vi "Save Moving Image.vi"() -> ()   [LabVIEW 2017]
uses:
  IMAQCV/PIIO/Core/PIIO DIO.ctl
  IMAQCV/GPIO/GPIO Pins.ctl
  <vilib>/Platform/TimedLoop/XDataNode/timing_clust.ctl
  <vilib>/Platform/TimedLoop/XDataNode/nitl_modes.ctl
  <vilib>/Platform/TimedLoop/XDataNode/wakeup.ctl
  <vilib>/platform/TimedLoop/XDataNode/XDataNode.xnode
  IMAQCV/PIIO.lvlib
  IMAQCV/IMAQCV.lvlib
  IMAQCV/LVOpenCV.lvlib
  <vilib>/Platform/TimedLoop/XDataNode/XDNodeRunTimeDep.lvlib
panel:
  in  "PIN":T1 items=["L1", "L2"]
  in  "delay (ms)":u32=150
  out "moving time (ms)":u32
  in  "LED Flash":bool
  in  "LED":bool
  in  "Gain (0=auto)":i32(slide) scale=0.0..100.0
  in  "Brightness":i32(slide)=50 scale=0.0..100.0
  in  "Contrast":i32(slide)=50 scale=0.0..100.0
  in  "Saturation":i32(slide)=50 scale=0.0..100.0
  in  "Sharpness":i32(slide)=50 scale=0.0..100.0
  in  "Rotation":i32(ring) items=["0", "90", "180", "270"]
  in  "Flip Horizontal":bool
  in  "Flip Vertical":bool
  in  "AWB":T2(ring)
  in  "Meter":enum16{"AVERAGE", "SPOT", "BACKLIT", "MATRIX"}(ring)
  in  "Effect":T3(ring)
  in  "Shutter (us, 0=auto)":i32
  out "output per minute":u32
  in  "File Format":string="camera-%03d.jpg"
  in  "Enable Save Files":bool
  in  "Image Index":u32
  in  "Image File Path":path=path "c:/project-01/camera-000.jpg"
  in  "FPS":i32=30
  in  "RGB LED 8x8":u32[][](array[colorbox])=[[0, 0, 16777215, 16777215, 16777215, 16777215, 16777215, 16777215], [0, 16777215, 16777215, 16777215, 16777215, 16777215, 16777215, 16777215], [16777215, 16777215, 16777215, 16777215, 16777215, 16777215, 16777215, 16777215], [16777215, 16777215, 0, 0, 0, 0, 0, 0], [16777215, 16777215, 0, 0, 0, 0, 0, 0], [16777215, 16777215, 0, 0, 0, 0, 0, 0], [16777215, 16777215, 0, 0, 0, 0, 0, 0], [0, 16777215, 16777215, 16777215, 16777215, 0, 0, 0]]
  in  "Image Size":T4(ring)=enum."640 (H)   x  480 (V) "
  out "picture":picture
  out "image processing time (ms)":u32
  out "DI-CH4":bool
  out "DI-CH2":bool
  out "DI-CH3":bool
  out "DI-CH1":bool
  in  "stop":bool
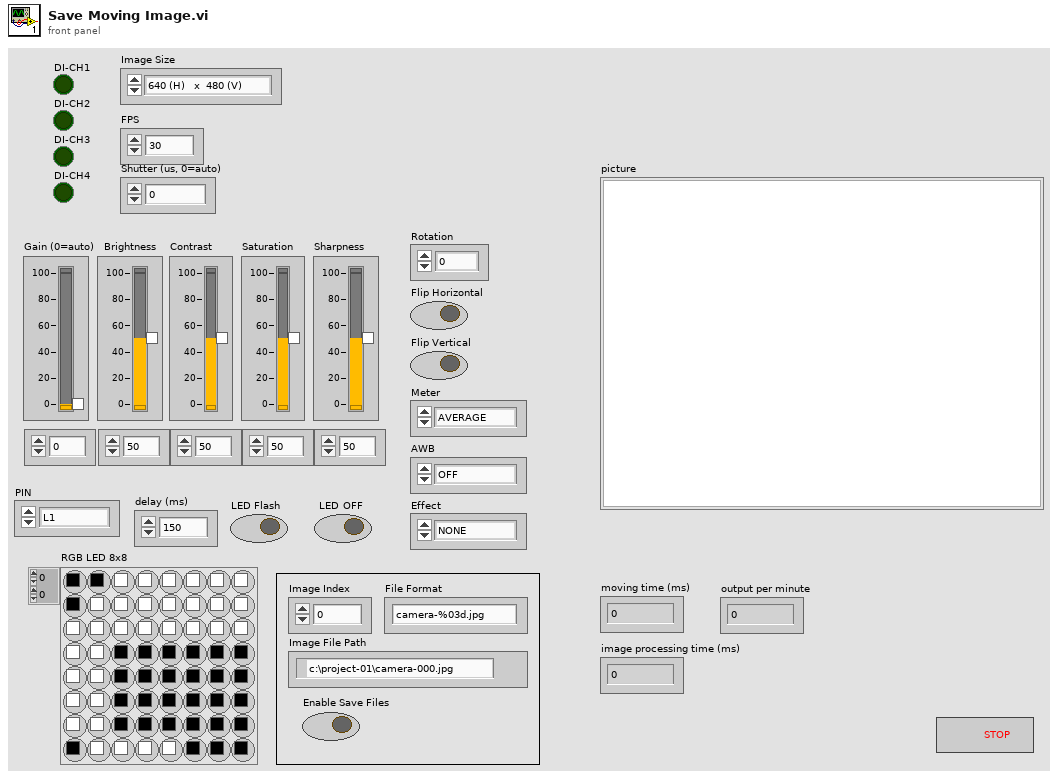
[diagram p1: front panel]
types:
  T1 = typedef "PIIO.lvlib/PIIO DIO.ctl" = u8
  T2 = enum16{"OFF", "AUTO", "SUNLIGHT", "CLOUDY", "SHADE", "TUNGSTEN", "FLUORESCENT", "INCANDESCENT", "FLASH"}
  T3 = enum16{"NONE", "NEGATIVE", "SOLARIZE", "SKETCH", "DENOISE", "EMBOSS", "OILPAINT", "HATCH", "GPEN", "PASTEL", "WATERCOLOR", "FILM", "BLUR", "SATURATION", "COLORSWAP", "WASHEDOUT", "POSTERISE", "COLORPOINT", "COLORBALANCE", "CARTOON"}
  T4 = enum16{"320 (H)   x  240 (V)", "352(H)    x  288 (V)", "640 (H)   x  480 (V) ", "800 (H)   x  600 (V)", "1024 (H) x  768 (V)", "1280 (H) x  720 (V)", "1280 (H) x  960 (V)", "1280 (H) x 1024 (V)", "1920 (H) x 1080 (V)"}
  T5 = typedef "PIIO.lvlib/GPIO Pins.ctl" = u8
  T6 = cluster{"GPIO":T5[], "MODE":enum8{"INPUT", "OUTPUT", "PWM_OUTPUT", "GPIO_CLOCK", "SOFT_PWM_OUTPUT", "SOFT_TONE_OUTPUT", "PWM_TONE_OUTPUT"}[]}
  T7 = typedef "Image Type" = u32
  T8 = typedef "IMAQCV.lvlib/IMAQCV Image.ctl" = refnum<vi>
  T9 = typedef "XDNodeRunTimeDep.lvlib/timing_clust.ctl" = cluster{"Expected End [f-1]":u64, "Actual End [f-1]":u64, "Finished Late? [f-1]":bool, "Expected End [i-1]":u64, "Actual End [i-1]":u64, "Finished Late? [i-1]":bool, "Expected Start [i]":u64, "Actual Start [i]":u64, "Expected Start [f]":u64, "Actual Start [f]":u64, "Source Name":string, "Structure Name":string, "Period":i64, "Deadline":i64, "Offset":i64, "Start":i64, "Priority":i32, "Timeout":i32, "Mode":T10, "Wakeup Reason":T11, "Error":errorcluster, "Source Type":string, "Secondary Source Type":string, "Global End Time":u64, "Global Start Time":u64, "Frame Duration":u64, "Iteration Duration":u64, "Assigned CPU":i32, "I/O Scan Engine Mode":u32}
  T10 = typedef "XDNodeRunTimeDep.lvlib/nitl_modes.ctl" = enum32{"No Change", "Process missed periods, maintain original phase", "Discard missed periods, maintain original phase", "Process missed periods, ignore original phase", "Discard missed periods, ignore original phase"}
  T11 = typedef "XDNodeRunTimeDep.lvlib/wakeup.ctl" = enum32{"Normal", "Aborted", "Asynchronous wakeup", "Timing source error", "Timed loop error", "Timeout"}
  T12 = typedef "IMAQ Image.ctl" = refnum<image>
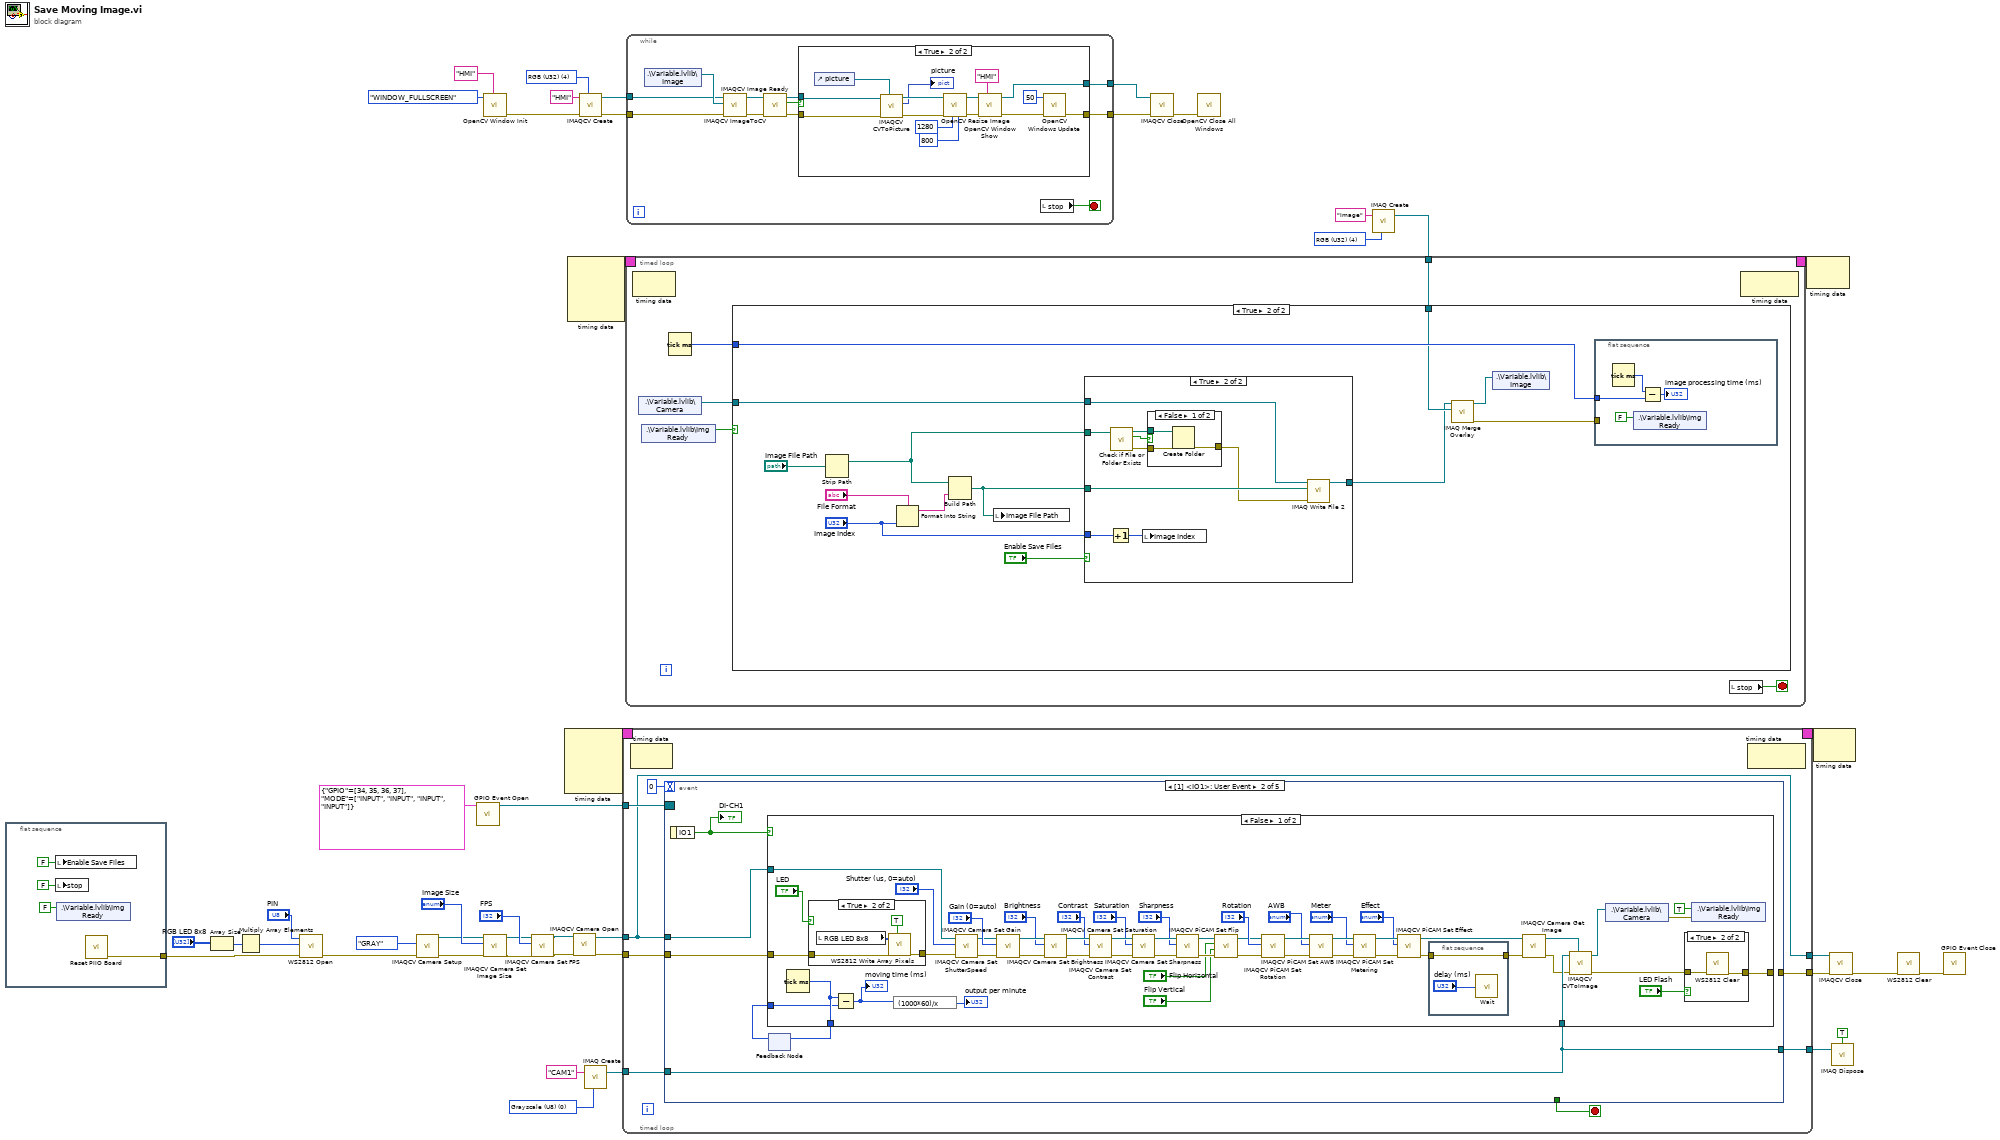
[diagram p0: block diagram]
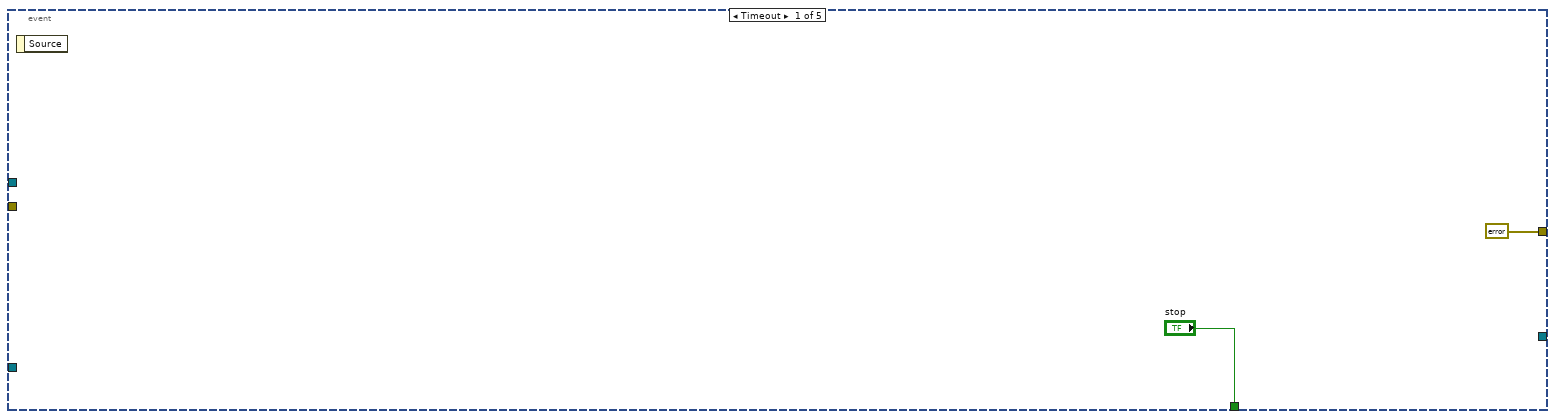
[diagram p6: hidden frame]
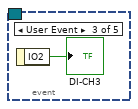
[diagram p10: hidden frame]
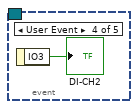
[diagram p11: hidden frame]
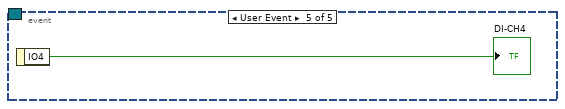
[diagram p12: hidden frame]
diagram:
  w20 = T7 4 items=["Grayscale (U8)", "Grayscale (I16)", "Grayscale (SGL)", "Complex (CSG)", "RGB (U32)", "HSL (U32)", "RGB (U64)", "Grayscale (U16)"] ("Image Type")
  w31 = u32 4 items=["Grayscale (U8)", "Grayscale (I16)", "Grayscale (SGL)", "Complex (CSG)", "RGB (U32)", "HSL (U32)", "RGB (U64)", "Grayscale (U16)"] ("Image Type")
  w36 = T7 0 items=["Grayscale (U8)", "Grayscale (I16)", "Grayscale (SGL)", "Complex (CSG)", "RGB (U32)", "HSL (U32)", "RGB (U64)", "Grayscale (U16)"] ("Image Type")
  n1 = flat-sequence {
    tunnel: [w47] -> w12
    frame #0 {
      n2 = local write "Enable Save Files"(FALSE ("Enable Save Files")) -> ()
      n3 = local write "stop"(FALSE ("stop")) -> ()
      n4 = shared-variable ".\\Variable.lvlib\\Img Ready"(FALSE ("outReady")) -> ()  [unwired: 1 in, 1 out]
      n5 = call "Reset PIIO Board.vi"() -> ("error out"=w47:errorcluster)  [unwired: 11 in]
    }
  }
  n6 = Array Size(array="RGB LED 8x8") -> (size(s)=w11:i32[])
  n7 = Multiply Array Elements(1:w11) -> (0:w9:i32)
  n8 = call "WS2812 Open.vi"("Error In"=w12, "Number of LEDs"=w9, "PIN"="PIN") -> ("Error Out"=w25:errorcluster)  [unwired: 8 in]
  n9 = call "IMAQCV Camera Setup.vi"("error in (no error)"=w25, "type"=enum16{"GRAY", "COLOR"}."GRAY") -> ("error out"=w26:errorcluster, "image out"=w27:T8)  [unwired: 8 in]
  n10 = call "GPIO Event Open.vi"("GPIO"=T6 {"GPIO"=[34, 35, 36, 37], "MODE"=[enum."INPUT", enum."INPUT", enum."INPUT", enum."INPUT"]}) -> ("Event Registration Refnum"=w13:refnum<event-registration>)  [unwired: 9 in, 1 out]
  n11 = call "OpenCV Window Init.vi"("window name"="HMI", "mode"=enum8{"WINDOW_AUTOSIZE", "WINDOW_FULLSCREEN"}."WINDOW_FULLSCREEN") -> ("error out"=w17:errorcluster)  [unwired: 9 in]
  n12 = call "IMAQCV Camera Set Image Size.vi"("error in (no error)"=w26, "Image Size"="Image Size", "image in"=w27) -> ("error out"=w8:errorcluster, "image out"=w7:T8)  [unwired: 7 in]
  n13 = call "IMAQCV Camera Set FPS.vi"("error in (no error)"=w8, "FPS"="FPS", "image in"=w7) -> ("error out"=w6:errorcluster, "image out"=w5:T8)  [unwired: 7 in]
  n14 = node-c288() -> (w45:T9)  [unwired: 4 in]
  n15 = node-c288() -> (w43:T9)  [unwired: 4 in]
  n16 = call "IMAQCV Camera Open.vi"("error in (no error)"=w6, "image in"=w5) -> ("error out"=w16:errorcluster, "image out"=w15:T8)  [unwired: 8 in]
  n17 = call "IMAQCV Create.vi"("Image Type"=w31, "error in (no error)"=w17, "Image Name"="HMI") -> ("error out"=w18:errorcluster, "Image Out"=w19:T8)  [unwired: 7 in]
  n18 = call "IMAQ Create"("Image Name"="CAM1", "Image Type"=w36) -> ("New Image"=w35:T12)  [unwired: 3 in, 1 out]
  n19 = timed-loop {
    tunnel: w13 -> [w55]
    tunnel: [w54] -> w40
    tunnel: w16 -> [w53]
    tunnel: w15 -> [w52]
    tunnel: [w52] -> w38
    tunnel: w35 -> [w51]
    timing: w45 -> [_]
    timing-out: [_] -> w44
    tunnel: [w50] -> w3
    stop <- w57 stop-if-true
    n20 = node-c288() -> ()  [unwired: 1 in, 1 out]
    n21 = event shown="[1] <IO1>: User Event" {
      selector: w55 -> [_ _ _ _ _]
      dyn-events: _ -> [_ _ _ _ _]
      timeout: 0 -> [_ _ _ _ _]
      tunnel: ["stop" _ _ _ _] -> w57
      tunnel: [errorcluster {"status"=FALSE, "code"=0, "source"=""} ("error out") _ _ _ _] -> w54
      tunnel: w52 -> [_ w64 _ _ _]
      tunnel: w53 -> [_ w65 _ _ _]
      tunnel: w51 -> [_ w63 _ _ _]
      tunnel: [_ w63 _ _ _] -> w50
      event Timeout {
        n22 = event-data() -> ()  [unwired: 1 in, 1 out]
      }
      event User Event {
        n23 = event-data() -> ("IO1"=w62:bool)  [unwired: 1 in]
        "DI-CH1" <- w62
        n24 = feedback #1() -> (w67:u32)  [unwired: 1 in]
        n25 = case shown="False" w62 {
          tunnel: w65 -> [w107 w131]
          tunnel: [w118 w131] -> _
          tunnel: w64 -> [w71 _]
          tunnel: w63 -> [w110 _]
          tunnel: w67 -> [w113 w130]
          tunnel: [w114 w130] -> w66
          frame False {
            n26 = Tick Count (ms)() -> (millisecond timer value=w114:u32)
            n27 = case shown="True" "LED" {
              tunnel: w107 -> [w120 w124]
              tunnel: [w120 w121] -> w73
              frame False {
              }
              frame True {
                n28 = local read "RGB LED 8x8"() -> (w122:u32[][])
                n29 = call "WS2812 Write Array Pixels.vi"("Refresh? (True)"=TRUE, "Error In"=w124, "pixmap"=w122) -> ("Error Out"=w121:errorcluster)  [unwired: 8 in]
              }
            }
            n30 = Subtract(x=w114, y=w113) -> (x-y=w69:u32)
            "moving time (ms)" <- w69
            n31 = expression code="(1000*60)/x"(w69) -> (→"output per minute":u32)
            n32 = call "IMAQCV Camera Set ShutterSpeed.vi"("error in (no error)"=w73, "shutter speed (us, 0=auto)"="Shutter (us, 0=auto)", "image in"=w71) -> ("error out"=w76:errorcluster, "image out"=w75:T8)  [unwired: 7 in]
            n33 = call "IMAQCV Camera Set Gain.vi"("error in (no error)"=w76, "gain (0=auto)"="Gain (0=auto)", "image in"=w75) -> ("error out"=w104:errorcluster, "image out"=w105:T8)  [unwired: 7 in]
            n34 = call "IMAQCV Camera Set Brightness.vi"("error in (no error)"=w104, "brightness"="Brightness", "image in"=w105) -> ("error out"=w103:errorcluster, "image out"=w100:T8)  [unwired: 7 in]
            n35 = call "IMAQCV Camera Set Contrast.vi"("error in (no error)"=w103, "contrast"="Contrast", "image in"=w100) -> ("error out"=w102:errorcluster, "image out"=w99:T8)  [unwired: 7 in]
            n36 = call "IMAQCV Camera Set Saturation.vi"("error in (no error)"=w102, "saturation"="Saturation", "image in"=w99) -> ("error out"=w101:errorcluster, "image out"=w98:T8)  [unwired: 7 in]
            n37 = call "IMAQCV Camera Set Sharpness.vi"("error in (no error)"=w101, "sharpness"="Sharpness", "image in"=w98) -> ("error out"=w91:errorcluster, "image out"=w90:T8)  [unwired: 7 in]
            n38 = call "IMAQCV PiCAM Set Flip.vi"("error in (no error)"=w91, "vertical"="Flip Vertical", "horizontal"="Flip Horizontal", "image in"=w90) -> ("error out"=w89:errorcluster, "image out"=w88:T8)  [unwired: 6 in]
            n39 = call "IMAQCV PiCAM Set Rotation.vi"("error in (no error)"=w89, "Rotation"="Rotation", "image in"=w88) -> ("error out"=w85:errorcluster, "image out"=w84:T8)  [unwired: 7 in]
            n40 = call "IMAQCV PiCAM Set AWB.vi"("error in (no error)"=w85, "AWB"="AWB", "image in"=w84) -> ("error out"=w82:errorcluster, "image out"=w80:T8)  [unwired: 7 in]
            n41 = call "IMAQCV PiCAM Set Metering.vi"("error in (no error)"=w82, "mode"="Meter", "image in"=w80) -> ("error out"=w81:errorcluster, "image out"=w79:T8)  [unwired: 7 in]
            n42 = call "IMAQCV PiCAM Set Effect.vi"("error in (no error)"=w81, "effect"="Effect", "image in"=w79) -> ("error out"=w72:errorcluster, "image out"=w70:T8)  [unwired: 7 in]
            n43 = flat-sequence {
              tunnel: [w128] -> w119
              tunnel: w72 -> [w128]
              frame #0 {
                n44 = call "Wait"("Count(mSec)"="delay (ms)") -> ()  [unwired: 1 out]
              }
            }
            n45 = call "IMAQCV Camera Get Image.vi"("error in (no error)"=w119, "image in"=w70) -> ("error out"=w109:errorcluster, "image out"=w108:T8)  [unwired: 8 in]
            n46 = call "IMAQCV CVToImage.vi"("cvimage in"=w108, "error in (no error)"=w109, "Variant In"=w110) -> ("error out"=w115:errorcluster, "Variant Out"=w111:refnum<image>)  [unwired: 7 in]
            n47 = shared-variable ".\\Variable.lvlib\\Camera"(w111) -> (error out=w116:errorcluster)  [unwired: 1 in]
            n48 = case shown="True" "LED Flash" {
              tunnel: [w125 w127] -> w118
              tunnel: w115 -> [w125 w126]
              frame False {
              }
              frame True {
                n49 = call "WS2812 Clear.vi"("Error In"=w126) -> ("Error Out"=w127:errorcluster)  [unwired: 10 in]
              }
            }
            n50 = shared-variable ".\\Variable.lvlib\\Img Ready"(TRUE ("ready"), error in=w116) -> ()  [unwired: 1 out]
          }
          frame True {
          }
        }
        n51 = feedback-in #1(w66) -> ()
      }
      event User Event {
        n52 = event-data() -> ("IO2"=→"DI-CH3":bool)  [unwired: 1 in]
      }
      event User Event {
        n53 = event-data() -> ("IO3"=→"DI-CH2":bool)  [unwired: 1 in]
      }
      event User Event {
        n54 = event-data() -> ("IO4"=→"DI-CH4":bool)  [unwired: 1 in]
      }
    }
    n55 = node-c288() -> ()  [unwired: 1 in, 1 out]
  }
  n56 = while {
    tunnel: [w144] -> w24
    tunnel: [w143] -> w23
    tunnel: w19 -> [w138]
    tunnel: w18 -> [w135]
    stop <- w145 stop-if-true
    n57 = shared-variable ".\\Variable.lvlib\\Image"() -> (w139:refnum<image>)  [unwired: 1 in, 1 out]
    n58 = call "IMAQCV ImageToCV.vi"("error in (no error)"=w135, "Variant In"=w139, "CV in"=w138) -> ("error out"=w136:errorcluster, "CV out"=w137:T8)  [unwired: 7 in]
    n59 = call "IMAQCV Image Ready.vi"("error in (no error)"=w136, "image in"=w137) -> ("error out"=w141:errorcluster, "ready?"=w140:bool, "image out"=w142:T8)  [unwired: 7 in]
    n60 = case shown="True" w140 {
      tunnel: [w146 w159] -> w144
      tunnel: [w147 w158] -> w143
      tunnel: w142 -> [w146 w150]
      tunnel: w141 -> [w147 w151]
      frame False {
      }
      frame True {
        n61 = control-ref of="picture"() -> (w149:refnum<vi>)
        n62 = call "IMAQCV CVToPicture.vi"("picture ref"=w149, "error in (no error)"=w151, "image"=w150) -> ("error out"=w152:errorcluster, "picture"=→"picture":picture, "image out"=w153:T8)  [unwired: 6 in]
        n63 = call "OpenCV Resize Image.vi"("height"=u32 800, "width"=u32 1280, "error in (no error)"=w152, "image in"=w153) -> ("error out"=w154:errorcluster, "image out"=w155:T8)  [unwired: 6 in]
        n64 = call "OpenCV Window Show.vi"("window name"="HMI", "error in (no error)"=w154, "image in"=w155) -> ("error out"=w160:errorcluster, "image out"=w159:T8)  [unwired: 7 in]
        n65 = call "OpenCV Windows Update.vi"("error in (no error)"=w160, "wait ms"=50) -> ("error out"=w158:errorcluster)  [unwired: 8 in, 1 out]
      }
    }
    n66 = local read "stop"() -> (w145:bool)
  }
  n67 = call "IMAQCV Close.vi"("error in (no error)"=w23, "Image"=w24) -> ("error out"=w33:errorcluster)  [unwired: 9 in]
  n68 = call "OpenCV Close All Windows.vi"("error in (no error)"=w33) -> ()  [unwired: 10 in, 1 out]
  n69 = call "IMAQ Create"("Image Name"="Image", "Image Type"=w20) -> ("New Image"=w4:T12)  [unwired: 3 in, 1 out]
  n70 = timed-loop {
    timing: w43 -> [_]
    timing-out: [_] -> w42
    tunnel: w4 -> [w163]
    stop <- w167 stop-if-true
    n71 = node-c288() -> ()  [unwired: 1 in, 1 out]
    n72 = shared-variable ".\\Variable.lvlib\\Camera"() -> (w165:refnum<image>)  [unwired: 1 in, 1 out]
    n73 = shared-variable ".\\Variable.lvlib\\Img Ready"() -> (w164:bool)  [unwired: 1 in, 1 out]
    n74 = Tick Count (ms)() -> (millisecond timer value=w166:u32)
    n75 = case shown="True" w164 {
      tunnel: w166 -> [_ w182]
      tunnel: w165 -> [_ w175]
      tunnel: w163 -> [_ w181]
      frame False {
      }
      frame True {
        n76 = Strip Path(path="Image File Path") -> (stripped path=w172:path)  [unwired: 1 out]
        n77 = Format Into String(format string="File Format", "Image Index") -> (resulting string=w176:string)  [unwired: 2 in, 1 out]
        n78 = Build Path(base path=w172, name or relative path=w176) -> (appended path=w171:path)
        n79 = local write "Image File Path"(w171) -> ()
        n80 = case shown="True" "Enable Save Files" {
          tunnel: w171 -> [_ w189]
          tunnel: w172 -> [_ w193]
          tunnel: "Image Index" -> [_ w188]
          tunnel: w175 -> [w183 w184]
          tunnel: [w183 w187] -> w174
          frame False {
          }
          frame True {
            n81 = Increment(x=w188) -> (x+1=w186:u32)
            n82 = call <vilib>:"Check if File or Folder Exists.vi"("path"=w193) -> ("error out"=w190:errorcluster, "file or folder exists?"=w192:bool, "dup path"=w191:path)  [unwired: 8 in]
            n83 = local write "Image Index"(w186) -> ()
            n84 = case shown="False" w192 {
              tunnel: w191 -> [w196 _]
              tunnel: w190 -> [w195 w197]
              tunnel: [w194 w197] -> w185
              frame False {
                n85 = Create Folder(path (use dialog)=w196, error in=w195) -> (error out=w194:errorcluster)  [unwired: 1 in, 2 out]
              }
              frame True {
              }
            }
            n86 = call-poly "IMAQ Write File 2"("error in (no error)"=w185, "File Path"=w189, "Image"=w184) -> ("Image Out (duplicate)"=w187:T12)  [unwired: 7 in, 1 out]
          }
        }
        n87 = call "IMAQ Merge Overlay"("Image Dst"=w181, "Image Src"=w174) -> ("error out"=w179:errorcluster, "Image Dst Out"=w180:T12)  [unwired: 8 in]
        n88 = shared-variable ".\\Variable.lvlib\\Image"(w180) -> ()  [unwired: 1 in, 1 out]
        n89 = flat-sequence {
          tunnel: w182 -> [w200]
          tunnel: w179 -> [_]
          frame #0 {
            n90 = Tick Count (ms)() -> (millisecond timer value=w201:u32)
            n91 = shared-variable ".\\Variable.lvlib\\Img Ready"(FALSE ("outReady")) -> ()  [unwired: 1 in, 1 out]
            n92 = Subtract(x=w201, y=w200) -> (x-y=→"image processing time (ms)":u32)
          }
        }
      }
    }
    n93 = local read "stop"() -> (w167:bool)
    n94 = node-c288() -> ()  [unwired: 1 in, 1 out]
  }
  n95 = node-c288(w42) -> ()  [unwired: 1 out]
  n96 = node-c288(w44) -> ()  [unwired: 1 out]
  n97 = call "IMAQCV Close.vi"("error in (no error)"=w40, "Image"=w38) -> ("error out"=w41:errorcluster)  [unwired: 9 in]
  n98 = call "IMAQ Dispose"("All Images? (No)"=TRUE, "Image"=w3) -> ()  [unwired: 4 in, 1 out]
  n99 = call "WS2812 Clear.vi"("Error In"=w41) -> ("Error Out"=w39:errorcluster)  [unwired: 10 in]
  n100 = call "GPIO Event Close.vi"("error in (no error)"=w39) -> ()  [unwired: 10 in, 1 out]
